vi "create Renderer.vi"(5 "pMaxTextureHeight":i32, 6 "pMaxTextureWidth":i32, 7 "pBytesPerVoxel":i32, 9 "pWindowHeight":i32, 10 "pWindowWidth":i32, 11 "pRendererId":i32) -> (3 "function return":i32)   [LabVIEW 2012, in "cvlib.lvlib"]
doc: "extern \"C\" __declspec(dllexport) long __cdecl createRenderer( long pRendererId,\n long pWindowWidth,\n long pWindowHeight,\n long pBytesPerVoxel,\n long pMaxTextureWidth,\n long pMaxTextureHeight);"
uses:
  cvlib.lvlib
  build/labview/lvcvlib/cvlib.dll
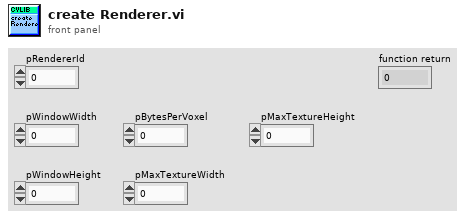
[diagram p1: front panel]
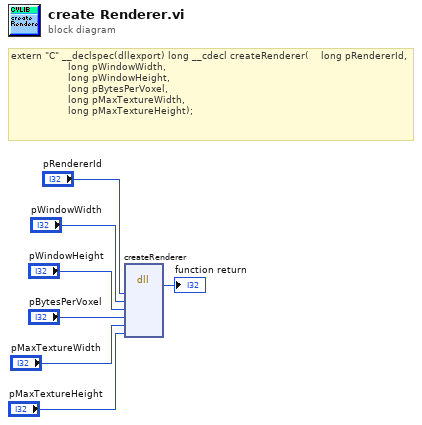
[diagram p0: block diagram]
diagram:
  # "extern \"C\" __declspec(dllexport) long __cdecl createRenderer(\t\t\t\tlong pRendererId,\n\t\t\t\t\t\t\t\t\t\t\t\t\t\t\t\t\t\t\tlong pWindowWidth,\n\t\t\t\t\t\t\t\t\t\t\t\t\t\t\t\t\t\t\tlong pWindowHeight,\n\t\t\t\t\t\t\t\t\t\t\t\t\t\t\t\t\t\t\tlong pBytesPerVoxel,\n\t\t\t\t\t\t\t\t\t\t\t\t\t\t\t\t\t\t\tlong pMaxTextureWidth,\n\t\t\t\t\t\t\t\t\t\t\t\t\t\t\t\t\t\t\tlong pMaxTextureHeight);"
  n1 = dll-call lib="C:/Users/myerslab/workspace2/Libraries/ClearVolume/build/labview/lvcvlib/cvlib.*" fn="createRenderer"("pRendererId"="pRendererId", "pWindowWidth"="pWindowWidth", "pWindowHeight"="pWindowHeight", "pBytesPerVoxel"="pBytesPerVoxel", "pMaxTextureWidth"="pMaxTextureWidth", "pMaxTextureHeight"="pMaxTextureHeight") -> (→"function return":i32)  [unwired: 9 in, 2 out]
